vi "Давление_код4_20.vi"(9 "Уставка давления":dbl(slide)=0.02 min=0.02 max=2.0 step=0.001 scale=0.0..1.0) -> (3 "mka":u16(slide)=4001 scale=4000.0..20000.0)   [LabVIEW 2018]
panel:
  in  "Мах.давление":dbl=1.0 min=0.0 max=20.299999237060547 step=9.999999747378752e-05
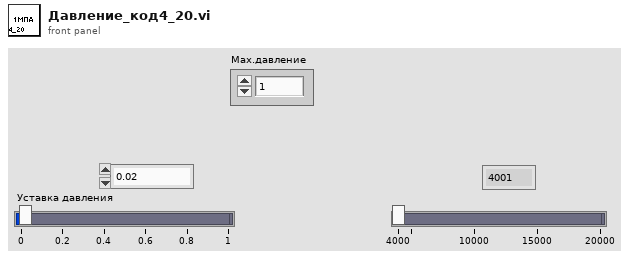
[diagram p1: front panel]
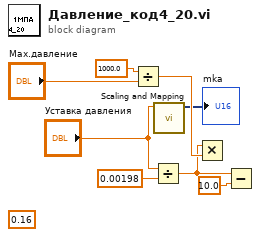
[diagram p0: block diagram]
diagram:
  (unwired) 0.16 ("y")
  n1 = Divide(x=1000.0, y="Мах.давление") -> (x/y=w7:dbl)
  n2 = Divide(x="Уставка давления", y=0.00198) -> (x/y=w3:dbl)
  n3 = call "Scaling and Mapping"("Signals"="Уставка давления") -> ("Scaled Signals"=→"mka":dynamicdata)  [unwired: 9 in, 1 out]
  n4 = Multiply(x=w3, y=w7) -> ()  [unwired: 1 out]
  n5 = Subtract(x=w3, y=10.0) -> ()  [unwired: 1 out]
